vi "LcWebView_example_3.vi"() -> ()   [LabVIEW 2019, in "LcWebView.lvclass"]
doc: "Inject javascript arguments"
uses:
  LcWebView.lvclass
  D:/GitProjects/Public/GitHub/LcWebView/data/Microsoft.Web.WebView2.WinForms.dll
  data/Microsoft.Web.WebView2.WinForms.dll
panel:
  out "BrowserProcessId":u32
  out "Initialise Loops":i32
  out "Status Message":string
  out "Status":i32(ring) items=["Created", "WaitingForActivation", "WaitingToRun", "Running", "WaitingForChildrenToComplete", "RanToCompletion", "Canceled", "Faulted"]
  in  "stop":bool
  in  "Web":refnum<k24>(container)
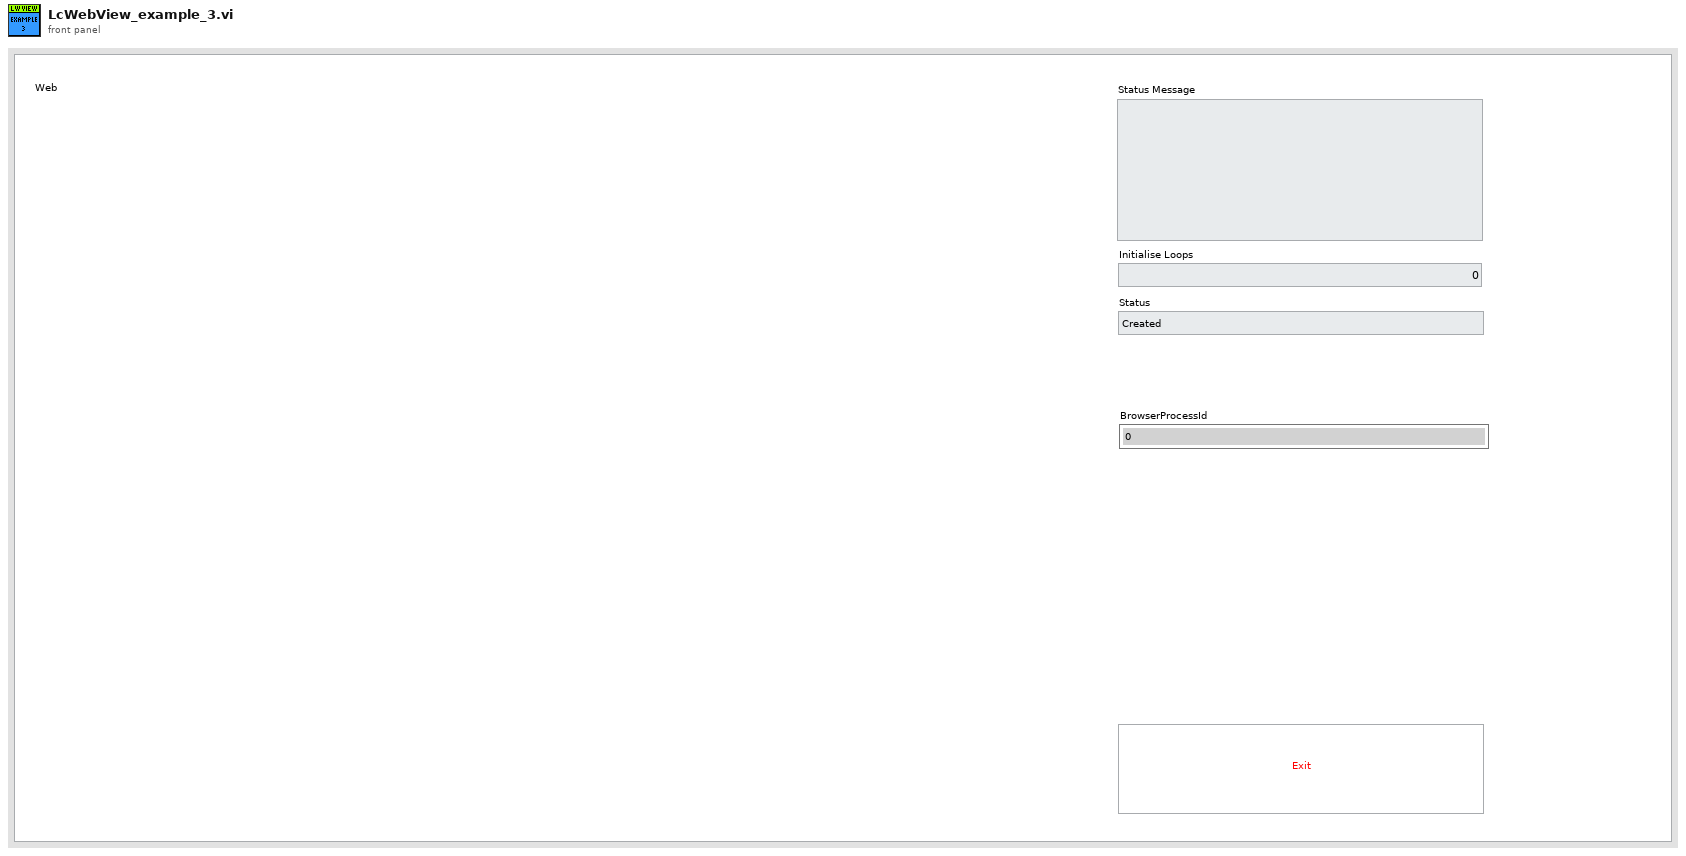
[diagram p1: front panel]
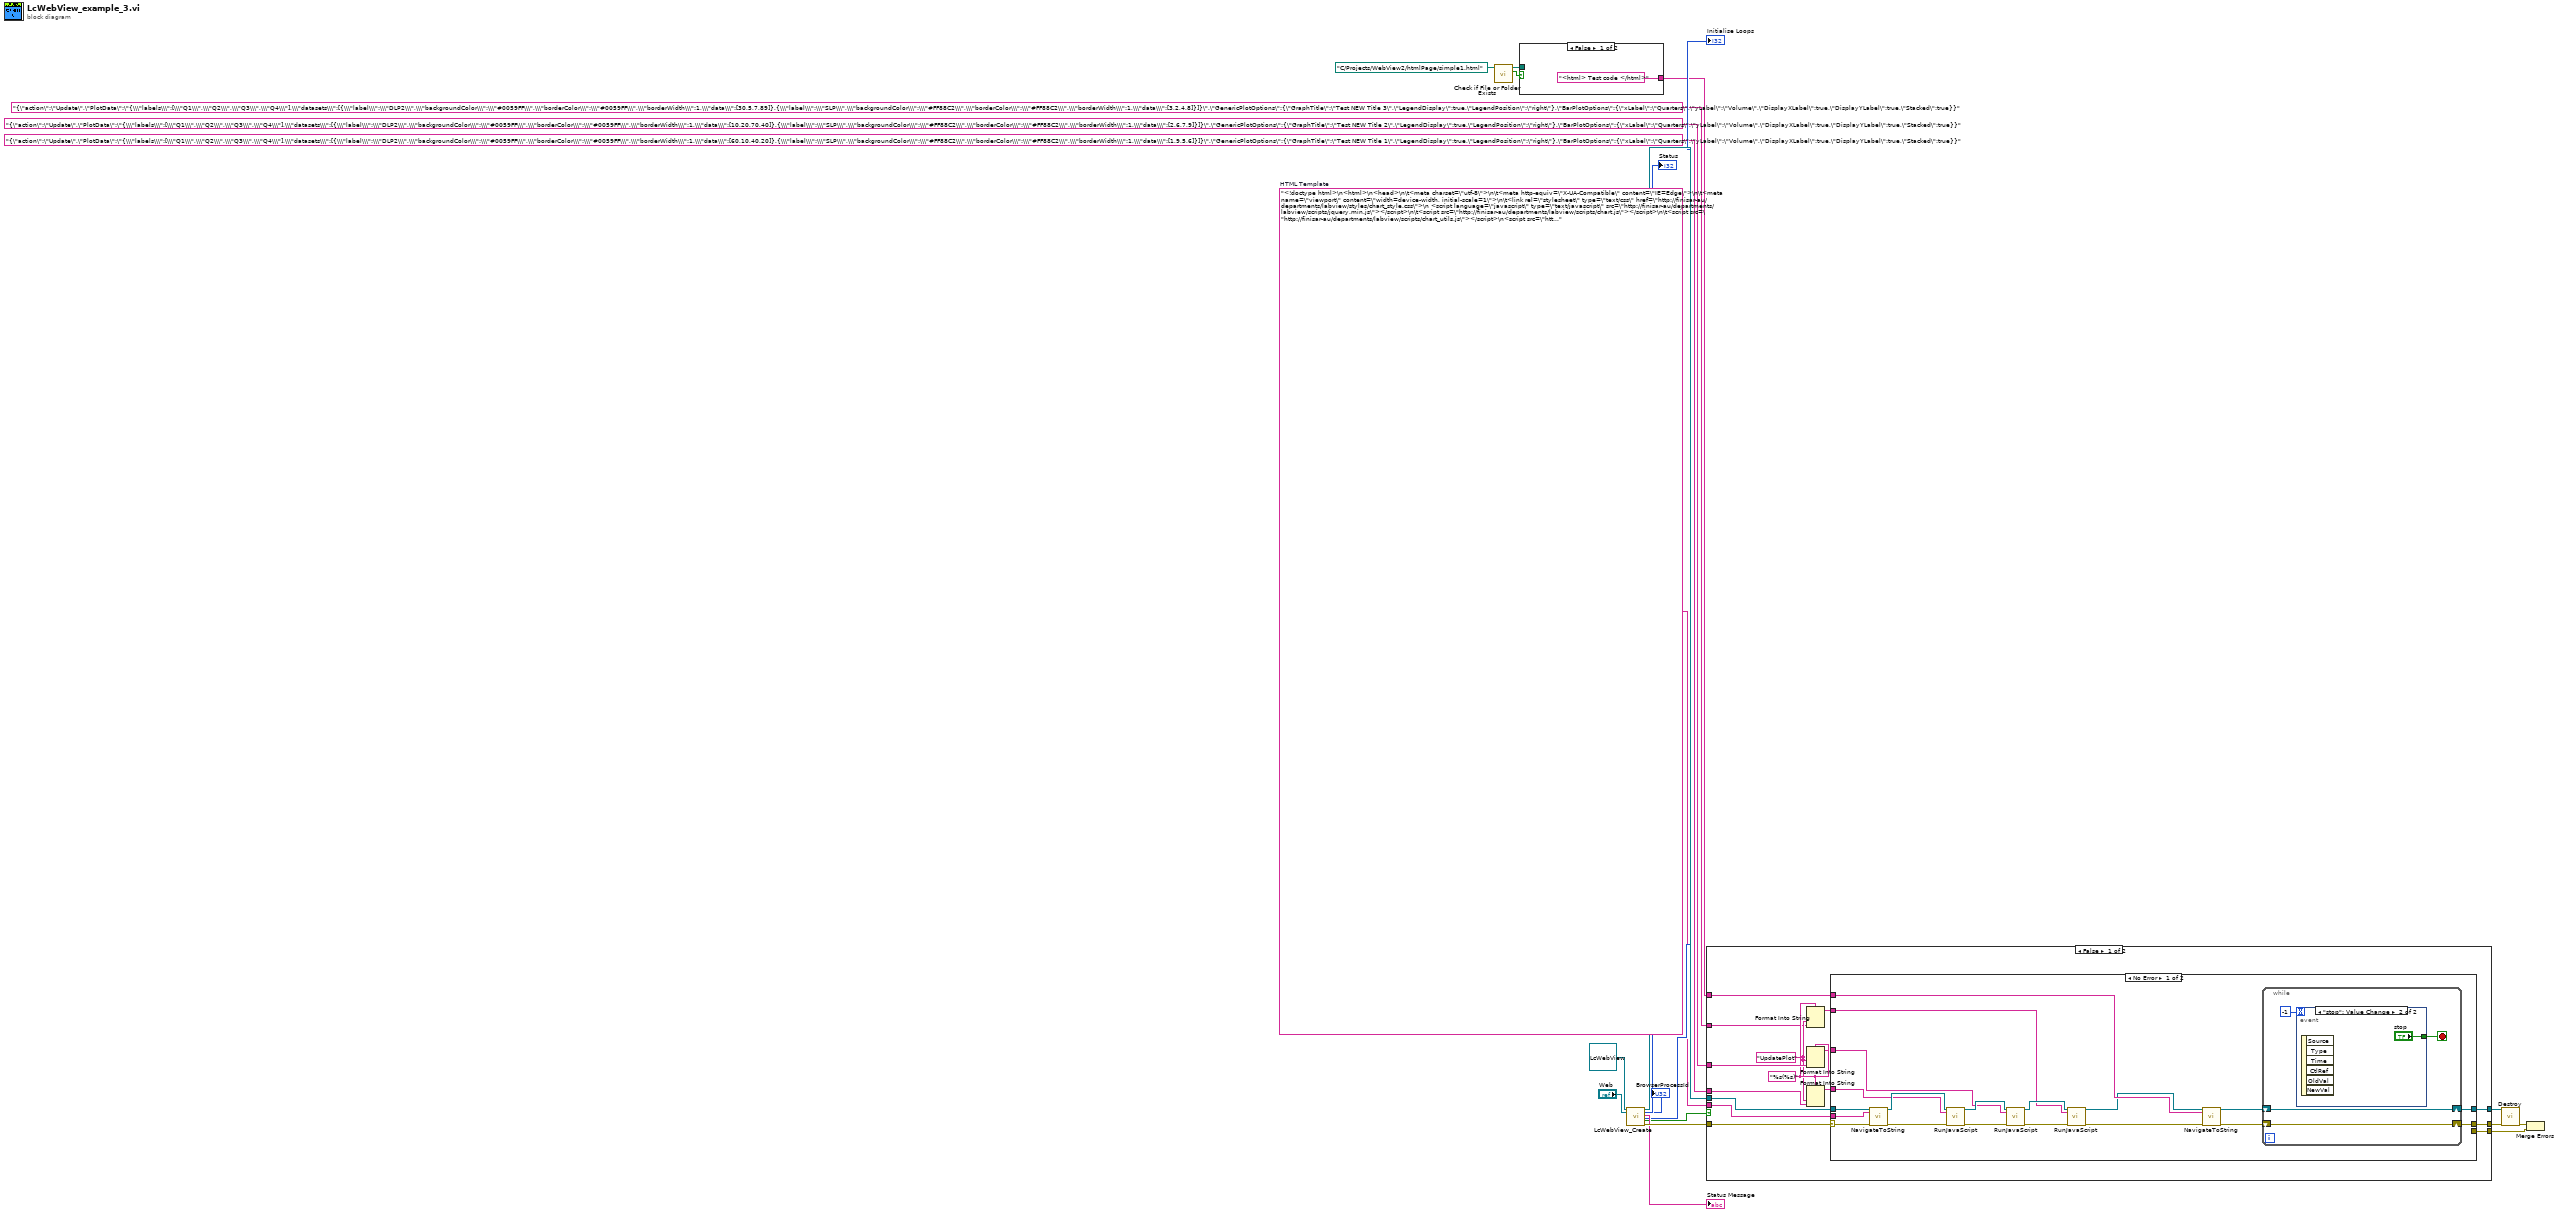
[diagram p0: block diagram]
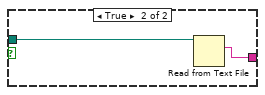
[diagram p2: hidden frame]
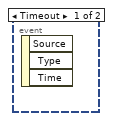
[diagram p3: hidden frame]
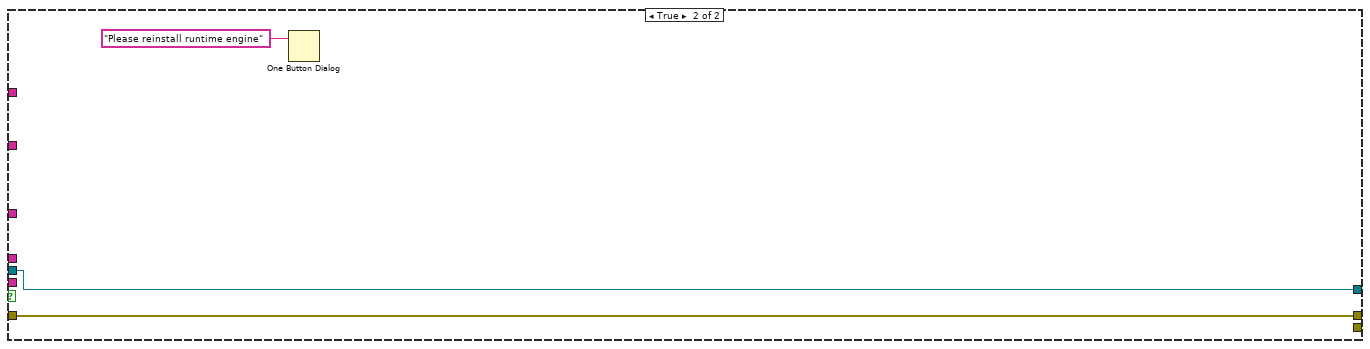
[diagram p5: hidden frame]
diagram:
  w9 = "<!doctype html>\n<html>\n<head>\n\t<meta charset=\"utf-8\">\n\t<meta http-equiv=\"X-UA-Compatible\" content=\"IE=Edge\">\n\t<meta name=\"viewport\" content=\"width=device-width, initial-scale=1\">\n\t<link rel=\"stylesheet\" type=\"text/css\" href=\"http://finisar-au/departments/labview/styles/chart_style.css\">\n <script language=\"javascript\" type=\"text/javascript\" src=\"http://finisar-au/departments/labview/scripts/jquery.min.js\"></script>\n\t<script src=\"http://finisar-au/departments/labview/scripts/chart.js\"></script>\n\t<script src=\"http://finisar-au/departments/labview/scripts/chart_utils.js\"></script>\n<script src=\"http://finisar-au/departments/labview/scripts/json2.js\"></script>\n    <script src=\"http://finisar-au/departments/labview/scripts/jquery(v1.11.3).min.js\"></script>\n    <style>\n    \t#container{\n            width:95vm;\n            height:95vh;\n            }\n        #canvas {\n\t\t-moz-user-select: none;\n\t\t-webkit-user-select: none;\n\t\t-ms-user-select: none;  \n\t   }\n\t    </style>\n</head>\n\n<body>\n<div id=\"container\">\n\t\t<canvas id=\"canvas\"></canvas>\n\t</div>\n\t<script type=\"text/javascript\">\n//---colour helper\nvar color = Chart.helpers.color;\nvar plotData ={}  \n\n // summarise config here --------------------------                   \n        var config = {\n\n// **************** PLOT TYPE***************************\n\t\t\ttype: 'bar',\n\n\t\t\tdata: plotData,\n//\t\t\t **************** PLOT OPTIONS : THIS PART WILL BE PLOT TYPE DEPENDENT***************************\noptions: \n{\nresponsive: true,\nmaintainAspectRatio: false,\n\t\t\t\tanimation: {\n\t\t\t\t\tanimateScale: true,\n\t\t\t\t\tanimateRotate: true\n\t\t\t\t},\nlegend: {\ndisplay:false,\t\t\t\t\t\t\nposition: 'right'\n\t\t\t\t\t},\ntitle: {\n\t\t\t\t\t\tdisplay:true,\n\t\t\t\t\t\ttext: 'INPUT'\n\t\t\t\t\t},  \n//*************************  ADDITIONAL OPTIONS   ***********************\n\t\t\t\tscales: {\n\t\t\t\t\txAxes: [{\n\t\t\t\t\t\t\tscaleLabel: {\n\t\t\t\t\t\t\tdisplay: true,\n\t\t\t\t\t\t\tlabelString: 'INPUT',\n       stacked:true\n\t\t\t\t\t\t}\n\t\t\t\t\t}],\n\t\t\t\t\tyAxes: [{\n\tticks: {\n\t\t\t\t\t\t\tmin: 0\n\t\t\t\t\t\t\t\t\t\t\t\t\t},\n\t\t\t\t\t\tscaleLabel: {\n\t\t\t\t\t\t\tdisplay: true,\n\t\t\t\t\t\t\tlabelString: 'INPUT',\n       stacked:true\n       \t\t\t\t\t\t}\n\t\t\t\t\t}]\n\t\t\t\t},\ntooltips: {\nenabled: true}\t\n}\n\t\t};\n\n// run plot function here -------------------------- \nwindow.onload = function() {\n\t  var ctx = document.getElementById('canvas').getContext('2d');\n\t\t\twindow.myChart = new Chart(ctx, config); \n};\n\nfunction UpdatePlot(data) {        \n    var myData = JSON.parse(data.PlotData);\n    config.data=myData;\n\tconfig.options.legend.display= data.GenericPlotOptions.LegendDisplay;\n\tconfig.options.legend.position=data.GenericPlotOptions.LegendPosition;            \n\tconfig.options.title.text=data.GenericPlotOptions.GraphTitle;\n\n//*************************  ADDITIONAL OPTIONS UPDATE ***********************\n\tconfig.options.scales.yAxes[0].stacked=data.BarPlotOptions.Stacked;\n\tconfig.options.scales.xAxes[0].stacked=data.BarPlotOptions.Stacked;\n\tconfig.options.scales.xAxes[0].scaleLabel.labelString=data.BarPlotOptions.xLabel;\n\tconfig.options.scales.yAxes[0].scaleLabel.labelString=data.BarPlotOptions.yLabel;\n\tconfig.options.scales.yAxes[0].scaleLabel.display=data.BarPlotOptions.DisplayYLabel;\n\tconfig.options.scales.xAxes[0].scaleLabel.display=data.BarPlotOptions.DisplayXLabel;\n\n//*************************  UPDATE PLOT ***********************\n\twindow.myChart.update();\n}\n\t</script>\n</body>\n</html>"  # HTML Template
  n1 = call <vilib>:"Check if File or Folder Exists.vi"("path"=path "C:/Projects/WebView2/htmlPage/simple1.html" ("DLLs path In")) -> ("file or folder exists?"=w5:bool, "dup path"=w4:path)  [unwired: 8 in, 1 out]
  n2 = case shown="False" w5 {
    tunnel: w4 -> [_ w24]
    tunnel: ["<html> Test code </html>" ("HTML Content") w23] -> w2
    frame False {
    }
    frame True {
      n3 = Read from Text File(file (use dialog)=w24) -> (text=w23:string)  [unwired: 3 in, 3 out]
    }
  }
  n4 = call "LcWebView_Create.vi"("reference in"=refnum<class "LcWebView.lvclass"> refnum, "Webview container"="Web") -> ("BrowserProcessId"=→"BrowserProcessId":u32, "reference out"=w19:refnum<class "LcWebView.lvclass">, "Status"=→"Status":i32, "Status Message"=→"Status Message":string, "Initialise Loops"=→"Initialise Loops":i32, "Reinstall Runtime"=w10:bool, "Error Out"=w18:errorcluster)  [unwired: 10 in, 1 out]
  n5 = case shown="False" w10 {
    tunnel: w19 -> [w39 w68]
    tunnel: w18 -> [w38 w67]
    tunnel: [w37 w68] -> w17
    tunnel: [w36 w67] -> w16
    tunnel: [w35 _] -> w11
    tunnel: w9 -> [w34 _]
    tunnel: "{\"action\":\"Update\",\"PlotData\":\"{\\\"labels\\\":[\\\"Q1\\\",\\\"Q2\\\",\\\"Q3\\\",\\\"Q4\\\"],\\\"datasets\\\":[{\\\"label\\\":\\\"DLP2\\\",\\\"backgroundColor\\\":\\\"#0059FF\\\",\\\"borderColor\\\":\\\"#0059FF\\\",\\\"borderWidth\\\":1,\\\"data\\\":[60,10,40,20]},{\\\"label\\\":\\\"SLP\\\",\\\"backgroundColor\\\":\\\"#FF88C2\\\",\\\"borderColor\\\":\\\"#FF88C2\\\",\\\"borderWidth\\\":1,\\\"data\\\":[1,9,5,6]}]}\",\"GenericPlotOptions\":{\"GraphTitle\":\"Test NEW Title 1\",\"LegendDisplay\":true,\"LegendPosition\":\"right\"},\"BarPlotOptions\":{\"xLabel\":\"Quarters\",\"yLabel\":\"Volume\",\"DisplayXLabel\":true,\"DisplayYLabel\":true,\"Stacked\":true}}" ("Java Script Function") -> [w33 _]
    tunnel: "{\"action\":\"Update\",\"PlotData\":\"{\\\"labels\\\":[\\\"Q1\\\",\\\"Q2\\\",\\\"Q3\\\",\\\"Q4\\\"],\\\"datasets\\\":[{\\\"label\\\":\\\"DLP2\\\",\\\"backgroundColor\\\":\\\"#0059FF\\\",\\\"borderColor\\\":\\\"#0059FF\\\",\\\"borderWidth\\\":1,\\\"data\\\":[10,20,70,40]},{\\\"label\\\":\\\"SLP\\\",\\\"backgroundColor\\\":\\\"#FF88C2\\\",\\\"borderColor\\\":\\\"#FF88C2\\\",\\\"borderWidth\\\":1,\\\"data\\\":[2,6,7,9]}]}\",\"GenericPlotOptions\":{\"GraphTitle\":\"Test NEW Title 2\",\"LegendDisplay\":true,\"LegendPosition\":\"right\"},\"BarPlotOptions\":{\"xLabel\":\"Quarters\",\"yLabel\":\"Volume\",\"DisplayXLabel\":true,\"DisplayYLabel\":true,\"Stacked\":true}}" ("Java Script Function") -> [w31 _]
    tunnel: "{\"action\":\"Update\",\"PlotData\":\"{\\\"labels\\\":[\\\"Q1\\\",\\\"Q2\\\",\\\"Q3\\\",\\\"Q4\\\"],\\\"datasets\\\":[{\\\"label\\\":\\\"DLP2\\\",\\\"backgroundColor\\\":\\\"#0059FF\\\",\\\"borderColor\\\":\\\"#0059FF\\\",\\\"borderWidth\\\":1,\\\"data\\\":[30,5,7,89]},{\\\"label\\\":\\\"SLP\\\",\\\"backgroundColor\\\":\\\"#FF88C2\\\",\\\"borderColor\\\":\\\"#FF88C2\\\",\\\"borderWidth\\\":1,\\\"data\\\":[3,2,4,8]}]}\",\"GenericPlotOptions\":{\"GraphTitle\":\"Test NEW Title 3\",\"LegendDisplay\":true,\"LegendPosition\":\"right\"},\"BarPlotOptions\":{\"xLabel\":\"Quarters\",\"yLabel\":\"Volume\",\"DisplayXLabel\":true,\"DisplayYLabel\":true,\"Stacked\":true}}" ("Java Script Function") -> [w28 _]
    tunnel: w2 -> [w25 _]
    frame False {
      w29 = "UpdatePlot" ("input 1")
      w30 = "%s(%s)" ("format string")
      n6 = Format Into String(format string=w30, w29, w28) -> (resulting string=w26:string)  [unwired: 2 in, 1 out]
      n7 = Format Into String(format string=w30, w29, w31) -> (resulting string=w27:string)  [unwired: 2 in, 1 out]
      n8 = Format Into String(format string=w30, w29, w33) -> (resulting string=w32:string)  [unwired: 2 in, 1 out]
      n9 = case shown="No Error" w38 {
        selector: w38 -> [w55 w64]
        tunnel: w39 -> [w56 w65]
        tunnel: [w58 w65] -> w37
        tunnel: [w57 _] -> w36
        tunnel: [_ w64] -> w35
        tunnel: w34 -> [w54 _]
        tunnel: w32 -> [w52 _]
        tunnel: w27 -> [w49 _]
        tunnel: w26 -> [w48 _]
        tunnel: w25 -> [w45 _]
        frame No Error {
          n10 = call-dynamic "NavigateToString.vi"("reference in"=w56, "HTML Content"=w54, "Error In"=w55) -> ("reference out"=w53:refnum<class "LcWebView.lvclass">, "Error Out"=w44:errorcluster)  [unwired: 14 in, 1 out]
          n11 = call-dynamic "RunJavaScript.vi"("reference in"=w53, "Java Script Function"=w52, "Error In"=w44) -> ("reference out"=w51:refnum<class "LcWebView.lvclass">, "Error Out"=w43:errorcluster)  [unwired: 13 in, 2 out]
          n12 = call-dynamic "RunJavaScript.vi"("reference in"=w51, "Java Script Function"=w49, "Error In"=w43) -> ("reference out"=w50:refnum<class "LcWebView.lvclass">, "Error Out"=w42:errorcluster)  [unwired: 13 in, 2 out]
          n13 = call-dynamic "RunJavaScript.vi"("reference in"=w50, "Java Script Function"=w48, "Error In"=w42) -> ("reference out"=w40:refnum<class "LcWebView.lvclass">, "Error Out"=w41:errorcluster)  [unwired: 13 in, 2 out]
          n14 = call-dynamic "NavigateToString.vi"("reference in"=w40, "HTML Content"=w45, "Error In"=w41) -> ("reference out"=w47:refnum<class "LcWebView.lvclass">, "Error Out"=w46:errorcluster)  [unwired: 14 in, 1 out]
          n15 = while {
            shift-right: [w62] -> w58
            shift-left: w47 -> [w62]
            shift-right: [w61] -> w57
            shift-left: w46 -> [w61]
            stop <- w59 stop-if-true
            n16 = event shown="[1] \"stop\": Value Change" {
              selector: _ -> [_ _]
              dyn-events: _ -> [_ _]
              timeout: -1 -> [_ _]
              tunnel: [_ "stop"] -> w59
              event Timeout {
                n17 = event-data() -> ()  [unwired: 1 in, 3 out]
              }
              event "stop": Value Change {
                n18 = event-data() -> ()  [unwired: 1 in, 6 out]
              }
            }
          }
        }
        frame Error {
        }
      }
    }
    frame True {
      n19 = One Button Dialog(message="Please reinstall runtime engine") -> ()  [unwired: 1 in, 1 out]
    }
  }
  n20 = call-dynamic "Destroy.vi"("reference in"=w17, "Error In"=w16) -> ("Error Out"=w15:errorcluster)  [unwired: 16 in, 1 out]
  n21 = Merge Errors(w15, w11) -> ()  [unwired: 1 out]
